vi "HEWH 50 Percent of First Draw.vi"(11 "Cold Gal Total Full\nData Set (Each Draw)":dbl[][](array[numeric])) -> (3 "Index Location":i32)   [LabVIEW 2023]
panel:
  out "Flow":dbl[](array[numeric])
  out "Search Value":dbl
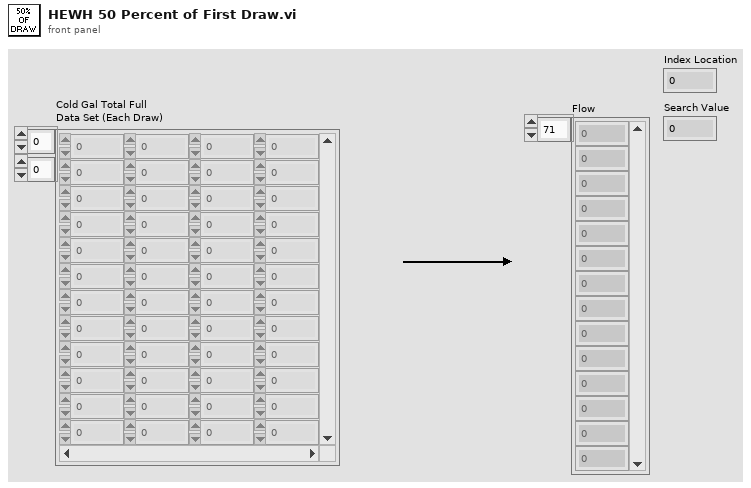
[diagram p1: front panel]
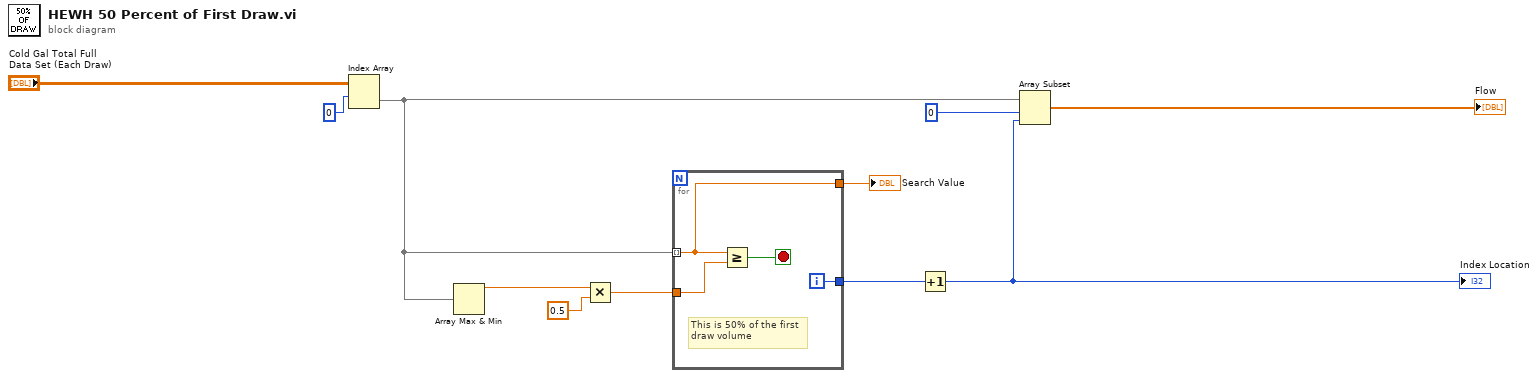
[diagram p0: block diagram]
diagram:
  n1 = Index Array "Index Array"(array="Cold Gal Total Full\nData Set (Each Draw)", index (row)=0) -> (element=w8:dbl[])  [unwired: 1 in]
  n2 = Array Max & Min(array=w8) -> (max value=w2:dbl)  [unwired: 3 out]
  n3 = Multiply(x=w2, y=0.5) -> (x*y=w4:dbl)
  n4 = for {
    tunnel: w4 -> [w15]
    tunnel: w8 -> [w12] mode=indexing
    tunnel: [w14] -> w10
    tunnel: [w12] -> w5
    i -> [w14]
    stop <- w13 stop-if-true
    # "This is 50% of the first\ndraw volume"
    n5 = Greater Or Equal?(x=w12, y=w15) -> (x >= y?=w13:bool)
  }
  "Search Value" <- w5
  n6 = Increment(x=w10) -> (x+1=w11:i32)
  "Index Location" <- w11
  n7 = Array Subset "Array Subset"(array=w8, index=0, length=w11) -> (→"Flow":dbl[])
